vi "19052 PreSet_AUTO_RANGE.vi"(8 "error in (no error)":errorcluster, 10 "on/off":u16(ring) items=["OFF", "ON"], 11 "VISA resource in":refnum<visa-resource-name>) -> (0 "error out":errorcluster, 2 "output command":string, 3 "VISA resource out":refnum<visa-resource-name>)   [LabVIEW 2015]
doc: "This VI writes to the instrument the AUTO RANGE state."
panel:
  # "PreSet Withstand voltage AUTO RANGE"
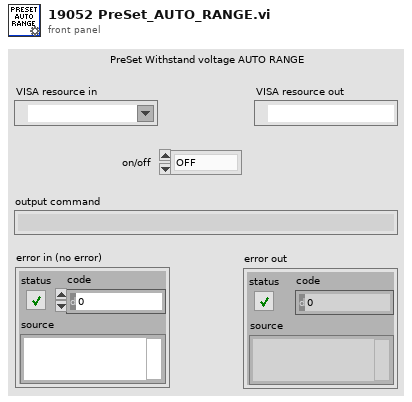
[diagram p1: front panel]
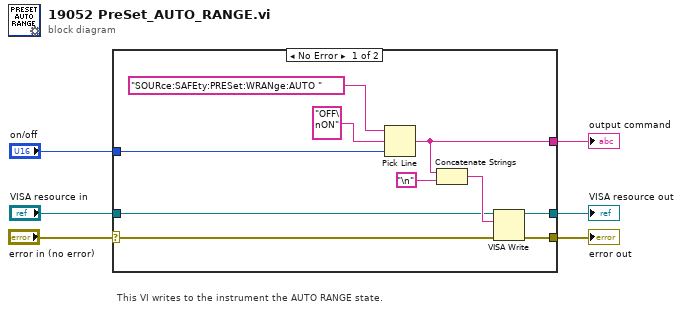
[diagram p0: block diagram]
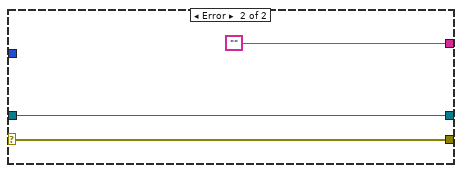
[diagram p2: hidden frame]
diagram:
  # "This VI writes to the instrument the AUTO RANGE state."
  n1 = case shown="No Error" "error in (no error)" {
    selector: "error in (no error)" -> [w15 w19]
    tunnel: [w16 w19] -> w6
    tunnel: [w10 w17] -> w4
    tunnel: [w9 ""] -> w3
    tunnel: "on/off" -> [w8 _]
    tunnel: "VISA resource in" -> [w7 w17]
    frame No Error {
      n2 = Pick Line(string ("")="SOURce:SAFEty:PRESet:WRANge:AUTO ", multi-line string="OFF\nON", line index=w8) -> (output string=w9:string)
      n3 = Concatenate Strings(w9, "\n") -> (w13:string)
      n4 = VISA Write(VISA resource name=w7, write buffer=w13, error in (no error)=w15) -> (VISA resource name out=w10:refnum<visa-resource-name>, error out=w16:errorcluster)  [unwired: 1 out]
    }
    frame Error {
    }
  }
  "error out" <- w6
  "VISA resource out" <- w4
  "output command" <- w3
